vi "AlliGator Register Control Events.vi"(8 "Error In":errorcluster, 11 "AlliGator Control References":T1) -> (0 "Error Out":errorcluster, 3 "AlliGator Event Registration":T2)   [LabVIEW 2021, in "AlliGator GUI.lvlib"]
doc: "Registers user events for controls on the main AlliGator window."
uses:
  AlliGator GUI.lvlib
  AlliGator Event Registration v2.ctl
  AlliGator Settings Event.ctl
  AlliGator Settings Window Messages.ctl
  AlliGator Phasor Color Map User Event List.ctl
  AlliGator Registered Events Ctrl Refnums.ctl
  Graphs/XY Graph/XY Graph Add-Ons.lvlib
  AlliGator Settings.lvlib
  AlliGator Phasor Plot Color Map.lvlib
  AlliGator Phasor Plot.lvlib
panel:
  # "see the AlliGator License on the block diagram (Ctrl+E or Window:Show Block Diagram)"
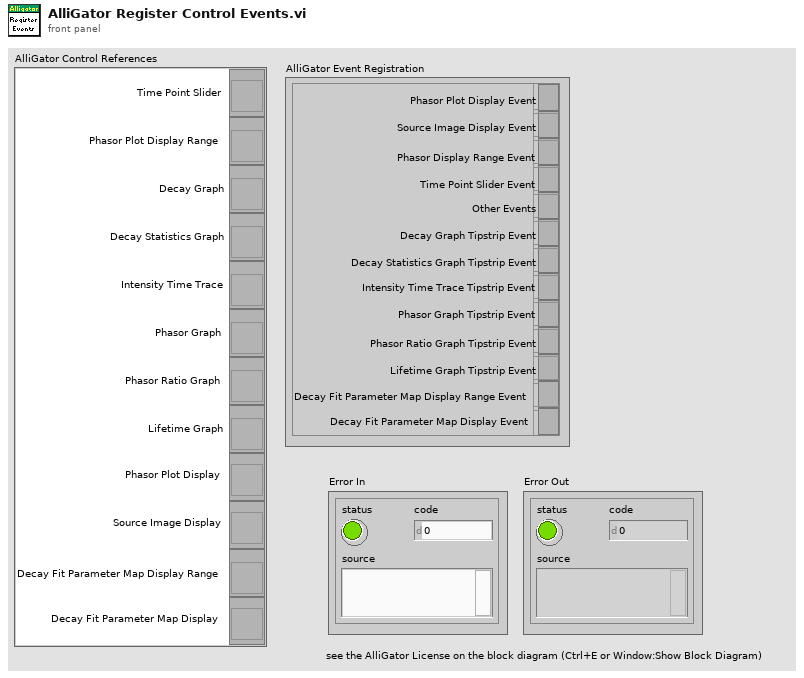
[diagram p1: front panel]
types:
  T1 = typedef "AlliGator GUI.lvlib/AlliGator Registered Events Ctrl Refnums.ctl" = cluster{"Time Point Slider":refnum<vi>, "Phasor Plot Display Range":refnum<vi>, "Decay Graph":refnum<vi>, "Decay Statistics Graph":refnum<vi>, "Intensity Time Trace":refnum<vi>, "Phasor Graph":refnum<vi>, "Phasor Ratio Graph":refnum<vi>, "Lifetime Graph":refnum<vi>, "Phasor Plot Display":refnum<vi>, "Source Image Display":refnum<vi>, "Decay Fit Parameter Map Display Range":refnum<vi>, "Decay Fit Parameter Map Display":refnum<vi>}
  T2 = typedef "AlliGator GUI.lvlib/AlliGator Event Registration v2.ctl" = cluster{"Phasor Plot Display Event":refnum<event-registration>, "Source Image Display Event":refnum<event-registration>, "Phasor Display Range Event":refnum<event-registration>, "Time Point Slider Event":refnum<event-registration>, "Other Events":refnum<event-registration>, "Decay Graph Tipstrip Event":refnum<event-registration>, "Decay Statistics Graph Tipstrip Event":refnum<event-registration>, "Intensity Time Trace Tipstrip Event":refnum<event-registration>, "Phasor Graph Tipstrip Event":refnum<event-registration>, "Phasor Ratio Graph Tipstrip Event":refnum<event-registration>, "Lifetime Graph Tipstrip Event":refnum<event-registration>, "Decay Fit Parameter Map Display Range Event":refnum<event-registration>, "Decay Fit Parameter Map Display Event":refnum<event-registration>}
  T3 = cluster{"Event Registration Refnum":refnum<event-registration>, "Event Registration Refnum":refnum<event-registration>, "Event Registration Refnum":refnum<event-registration>, "Event Registration Refnum":refnum<event-registration>, "Event Registration Refnum":refnum<event-registration>, "Event Registration Refnum":refnum<event-registration>, "Event Registration Refnum":refnum<event-registration>, "Event Registration Refnum":refnum<event-registration>, "Event Registration Refnum":refnum<event-registration>, "Event Registration Refnum":refnum<event-registration>, "Event Registration Refnum":refnum<event-registration>, "Event Registration Refnum":refnum<event-registration>, "Event Registration Refnum":refnum<event-registration>}
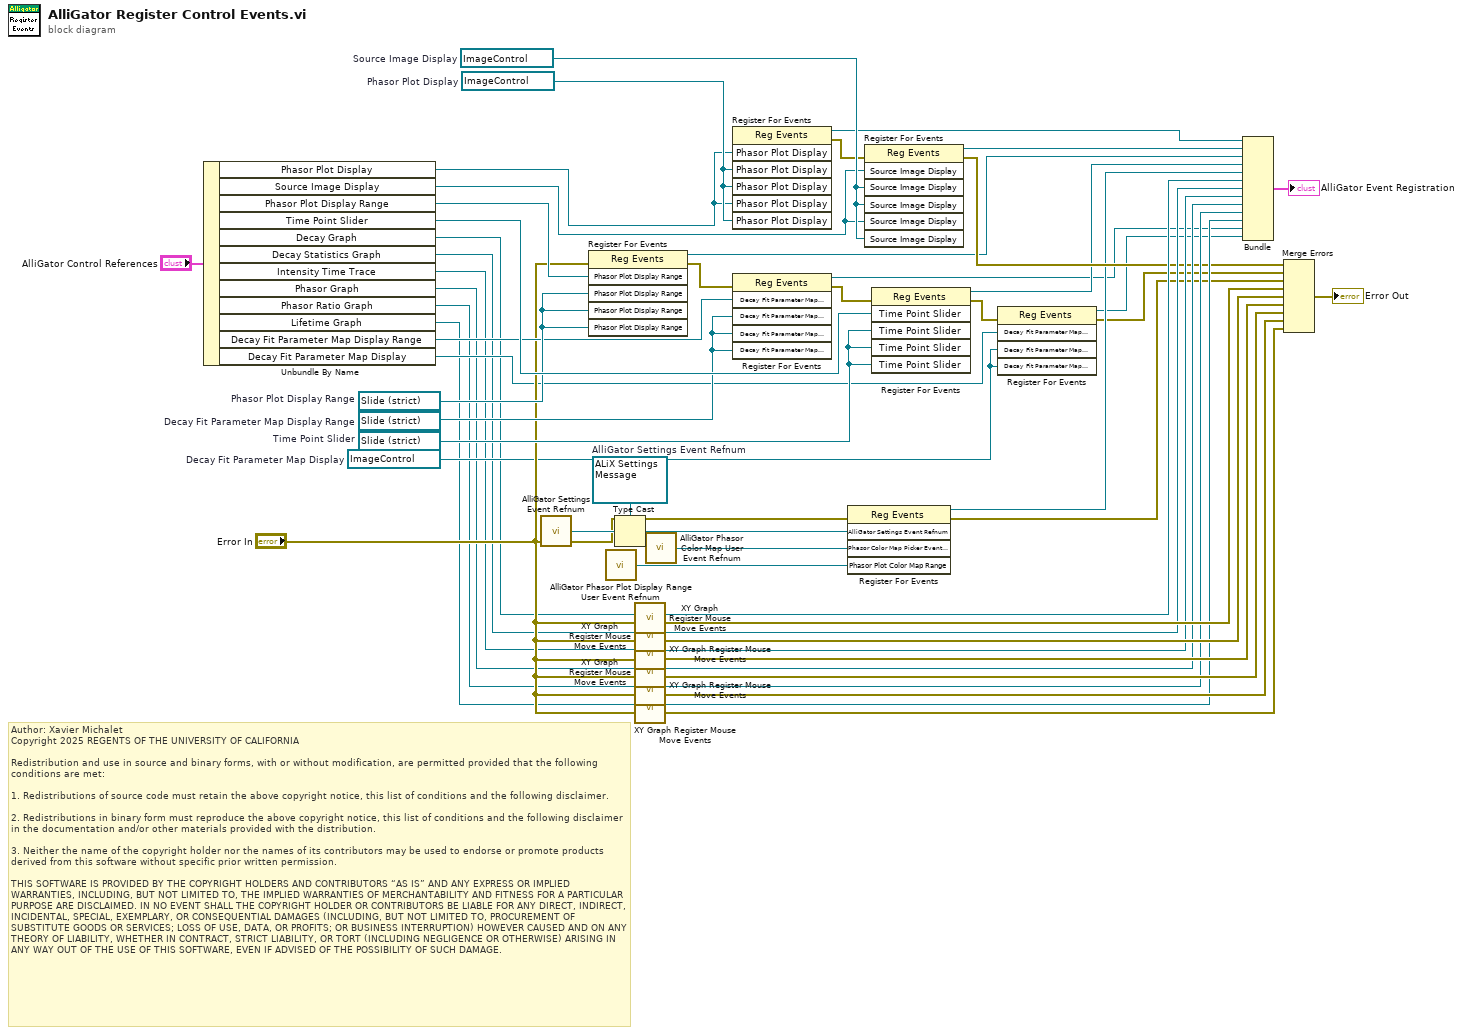
[diagram p0: block diagram]
diagram:
  w9 = refnum<vi> refnum  # Decay Fit Parameter Map Display
  w16 = refnum<vi> refnum  # Decay Fit Parameter Map Display Range
  w22 = refnum<vi> refnum  # Time Point Slider
  w23 = refnum<vi> refnum  # Phasor Plot Display Range
  w48 = refnum<user-event> refnum  # AlliGator Settings Event Refnum
  w37 = refnum<vi> refnum  # Source Image Display
  w38 = refnum<vi> refnum  # Phasor Plot Display
  # "Author: Xavier Michalet\nCopyright 2025 REGENTS OF THE UNIVERSITY OF CALIFORNIA\n\nRedistribution and use in source and binary forms, with or without modification, are permitted provided that the following conditions are met:\n\n1. Redistributions of source code must retain the above copyright notice, this list of conditions and the following disclaimer.\n\n2. Redistributions in binary form must reproduce the above copyright notice, this list of conditions and the following disclaimer in the documentation and/or other materials provided with the distribution.\n\n3. Neither the name of the copyright holder nor the names of its contributors may be used to endorse or promote products derived from this software without specific prior written permission.\n\nTHIS SOFTWARE IS PROVIDED BY THE COPYRIGHT HOLDERS AND CONTRIBUTORS “AS IS” AND ANY EXPRESS OR IMPLIED WARRANTIES, INCLUDING, BUT NOT LIMITED TO, THE IMPLIED WARRANTIES OF MERCHANTABILITY AND FITNESS FOR A PARTICULAR PURPOSE ARE DISCLAIMED. IN NO EVENT SHALL THE COPYRIGHT HOLDER OR CONTRIBUTORS BE LIABLE FOR ANY DIRECT, INDIRECT, INCIDENTAL, SPECIAL, EXEMPLARY, OR CONSEQUENTIAL DAMAGES (INCLUDING, BUT NOT LIMITED TO, PROCUREMENT OF SUBSTITUTE GOODS OR SERVICES; LOSS OF USE, DATA, OR PROFITS; OR BUSINESS INTERRUPTION) HOWEVER CAUSED AND ON ANY THEORY OF LIABILITY, WHETHER IN CONTRACT, STRICT LIABILITY, OR TORT (INCLUDING NEGLIGENCE OR OTHERWISE) ARISING IN ANY WAY OUT OF THE USE OF THIS SOFTWARE, EVEN IF ADVISED OF THE POSSIBILITY OF SUCH DAMAGE."
  n1 = Unbundle By Name("AlliGator Control References") -> ("Phasor Plot Display"=w13:refnum<vi>, "Source Image Display"=w15:refnum<vi>, "Phasor Plot Display Range"=w27:refnum<vi>, "Time Point Slider"=w25:refnum<vi>, "Decay Graph"=w6:refnum<vi>, "Decay Statistics Graph"=w5:refnum<vi>, "Intensity Time Trace"=w4:refnum<vi>, "Phasor Graph"=w3:refnum<vi>, "Phasor Ratio Graph"=w2:refnum<vi>, "Lifetime Graph"=w1:refnum<vi>, "Decay Fit Parameter Map Display Range"=w20:refnum<vi>, "Decay Fit Parameter Map Display"=w10:refnum<vi>)
  n2 = call "AlliGator Settings Event Refnum.vi"("Error In"="Error In") -> ("AlliGator Settings Event Refnum"=w47:refnum<user-event>, "Error Out"=w21:errorcluster)  [unwired: 7 in]
  n3 = register-events(error in="Error In", w27, w23, w23, w23) -> (reference out=w26:refnum<event-registration>, error out=w19:errorcluster)  [unwired: 1 in]
  n4 = call "AlliGator Phasor Plot Display Range User Event Refnum.vi"() -> ("Phasor Plot Color Map Range"=w32:refnum<user-event>)  [unwired: 9 in]
  n5 = Type Cast(type=w48, x=w47) -> (*(type *) &x=w34:refnum<user-event>)
  n6 = call "XY Graph Register Mouse Move Events.vi"("Error In"="Error In", "XY Graph Refnum"=w6) -> ("Error Out"=w54:errorcluster, "Event Registration Refnum"=w41:refnum<event-registration>)  [unwired: 8 in]
  n7 = call "XY Graph Register Mouse Move Events.vi"("Error In"="Error In", "XY Graph Refnum"=w5) -> ("Error Out"=w53:errorcluster, "Event Registration Refnum"=w42:refnum<event-registration>)  [unwired: 8 in]
  n8 = call "XY Graph Register Mouse Move Events.vi"("Error In"="Error In", "XY Graph Refnum"=w4) -> ("Error Out"=w52:errorcluster, "Event Registration Refnum"=w43:refnum<event-registration>)  [unwired: 8 in]
  n9 = call "XY Graph Register Mouse Move Events.vi"("Error In"="Error In", "XY Graph Refnum"=w3) -> ("Error Out"=w51:errorcluster, "Event Registration Refnum"=w44:refnum<event-registration>)  [unwired: 8 in]
  n10 = call "XY Graph Register Mouse Move Events.vi"("Error In"="Error In", "XY Graph Refnum"=w2) -> ("Error Out"=w50:errorcluster, "Event Registration Refnum"=w45:refnum<event-registration>)  [unwired: 8 in]
  n11 = call "XY Graph Register Mouse Move Events.vi"("Error In"="Error In", "XY Graph Refnum"=w1) -> ("Error Out"=w49:errorcluster, "Event Registration Refnum"=w46:refnum<event-registration>)  [unwired: 8 in]
  n12 = call "AlliGator Phasor Color Map User Event Refnum.vi"() -> ("Phasor Color Map Picker Event Refnum"=w33:refnum<user-event>)  [unwired: 9 in]
  n13 = register-events(w13, w38, w38, w13, w38) -> (reference out=w36:refnum<event-registration>, error out=w29:errorcluster)  [unwired: 2 in]
  n14 = register-events(error in=w19, w20, w16, w16, w16) -> (reference out=w17:refnum<event-registration>, error out=w18:errorcluster)  [unwired: 1 in]
  n15 = register-events(error in=w21, w34, w33, w32) -> (reference out=w30:refnum<event-registration>, error out=w28:errorcluster)  [unwired: 1 in]
  n16 = register-events(error in=w29, w15, w37, w37, w15, w37) -> (reference out=w35:refnum<event-registration>, error out=w31:errorcluster)  [unwired: 1 in]
  n17 = register-events(error in=w18, w25, w22, w22, w22) -> (reference out=w24:refnum<event-registration>, error out=w12:errorcluster)  [unwired: 1 in]
  n18 = register-events(error in=w12, w10, w9, w9) -> (reference out=w8:refnum<event-registration>, error out=w11:errorcluster)  [unwired: 1 in]
  n19 = Bundle("Event Registration Refnum"=w36, "Event Registration Refnum"=w35, "Event Registration Refnum"=w26, "Event Registration Refnum"=w24, "Event Registration Refnum"=w30, "Event Registration Refnum"=w41, "Event Registration Refnum"=w42, "Event Registration Refnum"=w43, "Event Registration Refnum"=w44, "Event Registration Refnum"=w45, "Event Registration Refnum"=w46, "Event Registration Refnum"=w17, "Event Registration Refnum"=w8) -> (→"AlliGator Event Registration":T3)  [unwired: 1 in]
  n20 = Merge Errors(w31, w11, w28, w54, w53, w52, w51, w50, w49) -> (→"Error Out":errorcluster)
